vi "Test Folder--constant.vi"() -> (3 "Test Folder":path)   [LabVIEW 2025]
doc: "This constant contains the temporary testing directory."
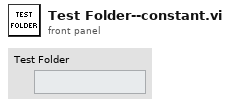
[diagram p1: front panel]
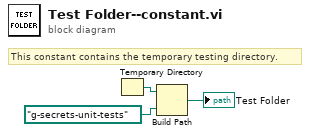
[diagram p0: block diagram]
diagram:
  # "This constant contains the temporary testing directory."
  n1 = Temporary Directory() -> (w3:path)
  n2 = Build Path(base path=w3, name or relative path=path "g-secrets-unit-tests" ("Test Folder")) -> (appended path=→"Test Folder":path)
